vi "simx Get Object Child.vi"(6 "operationMode":i32, 7 "childObjectHandle":i32, 8 "error in (no error)":errorcluster, 9 "childIndex":i32, 10 "parentObjectHandle":i32, 11 "clientID":i32) -> (0 "error out":errorcluster, 3 "function return":i32, 5 "childObjectHandle out":i32)   [LabVIEW 2019, in "PXL_V-REP.lvlib"]
doc: "EXTAPI_DLLEXPORT simxInt simxGetObjectChild(simxInt clientID,simxInt parentObjectHandle,simxInt childIndex,simxInt* childObjectHandle,simxInt operationMode);"
uses:
  PXL_V-REP.lvlib
  <userlib>/V-REP/remoteApi.dll
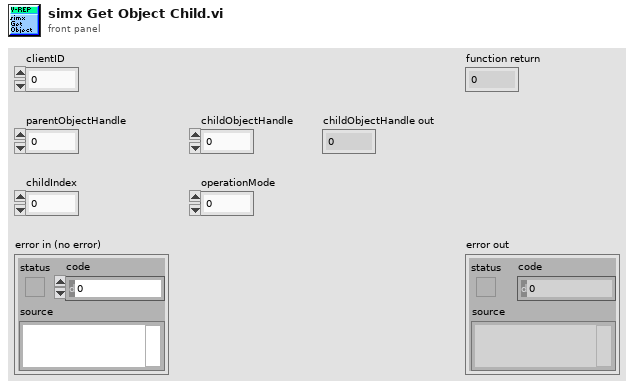
[diagram p1: front panel]
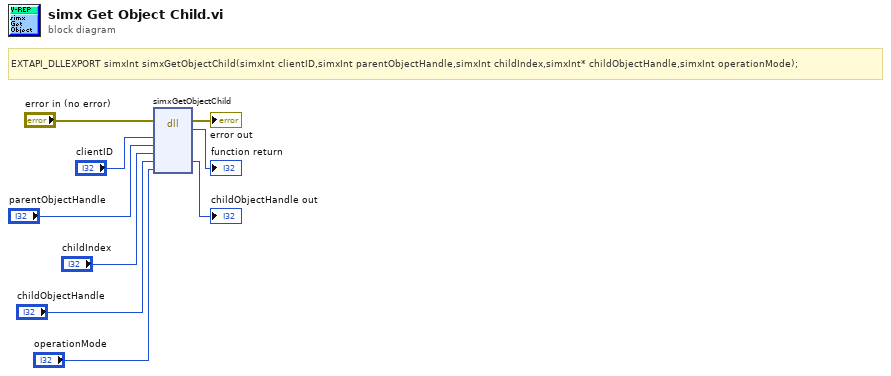
[diagram p0: block diagram]
diagram:
  # "EXTAPI_DLLEXPORT simxInt simxGetObjectChild(simxInt clientID,simxInt parentObjectHandle,simxInt childIndex,simxInt* childObjectHandle,simxInt operationMode);"
  n1 = dll-call lib="C:/Program Files (x86)/National Instruments/LabVIEW 2019/user.lib/V-REP/remoteApi.*" fn="simxGetObjectChild"(error in="error in (no error)", "clientID"="clientID", "parentObjectHandle"="parentObjectHandle", "childIndex"="childIndex", "childObjectHandle"="childObjectHandle", "operationMode"="operationMode") -> (error out=→"error out":errorcluster, →"function return":i32, "childObjectHandle"=→"childObjectHandle out":i32)  [unwired: 6 in, 1 out]
